vi "BNT_ULx-Content.vi"() -> (0 "CS++Classes & Messages":T1(array[cluster]))   [LabVIEW 2020]
doc: "Place actor and class constants that should be included included in the COMPACT application on the blockdiagramm."
uses:
  <vilib>/ActorFramework/Message/Message.lvclass
  BNT_ULx-MCSV/BNT_ULx-MCSV-I/BNT_ULx-MCSV-I/BNT_ULx-MCSV-I.lvclass
  C:/User/Brand/LVP/CSPP/CSPP-Template/Packages/CSPP_Core/Actors/CSPP_DeviceActor/CSPP_DeviceActor.lvclass
  CSPP_Core/Actors/CSPP_DeviceActor/CSPP_DeviceActor.lvclass
  C:/User/Brand/LVP/CSPP/CSPP-Template/Packages/CSPP_Core/Actors/CSPP_BaseActor/CSPP_BaseActor.lvclass
  CSPP_Core/Actors/CSPP_BaseActor/CSPP_BaseActor.lvclass
  BNT_ULx-MCSV/BNT_ULx-MCSV/BNT_ULx-MCSV.lvclass
  BNT_ULx-MCSV/BNT_ULx-MCSV-RTD/BNT_ULx-MCSV-RTD.lvclass
  BNT_ULx-MCSV/BNT_ULx-MCSV-TC/BNT_ULx-MCSV-TC.lvclass
  BNT_ULx-MCSV/BNT_ULx-MCSV-Ctr2Freq/BNT_ULx-MCSV-Ctr2Freq.lvclass
  BNT_ULx-MCSV/BNT_ULx-MCSV-DOPWM/BNT_ULx-MCSV-DOPWM.lvclass
  BNT_ULx-MCSV/BNT_ULx-MCSV-AIAvg/BNT_ULx-MCSV-AIAvg.lvclass
  C:/Program Files (x86)/National Instruments/LabVIEW 2020/vi.lib/ActorFramework/Actor/Actor.lvclass
  C:/User/Brand/LVP/CSPP/CSPP-Template/Packages/BNT_ULx/BNT_ULx-MCSV/BNT_ULx-MCSV/BNT_ULx-MCSV.lvclass
  C:/User/Brand/LVP/CSPP/CSPP-Template/Packages/BNT_ULx/BNT_ULx-MCSV/BNT_ULx-MCSV-RTD/BNT_ULx-MCSV-RTD.lvclass
  C:/User/Brand/LVP/CSPP/CSPP-Template/Packages/BNT_ULx/BNT_ULx-MCSV/BNT_ULx-MCSV-TC/BNT_ULx-MCSV-TC.lvclass
  C:/User/Brand/LVP/CSPP/CSPP-Template/Packages/BNT_ULx/BNT_ULx-MCSV/BNT_ULx-MCSV-Ctr2Freq/BNT_ULx-MCSV-Ctr2Freq.lvclass
  C:/User/Brand/LVP/CSPP/CSPP-Template/Packages/BNT_ULx/BNT_ULx-MCSV/BNT_ULx-MCSV-DOPWM/BNT_ULx-MCSV-DOPWM.lvclass
  C:/User/Brand/LVP/CSPP/CSPP-Template/Packages/BNT_ULx/BNT_ULx-MCSV/BNT_ULx-MCSV-AIAvg/BNT_ULx-MCSV-AIAvg.lvclass
  C:/User/Brand/LVP/CSPP/CSPP-Template/Packages/BNT_ULx/BNT_ULx-MCSV/BNT_ULx-MCSV-I/BNT_ULx-MCSV-I/BNT_ULx-MCSV-I.lvclass
panel:
  # "Place actor and class constants on the blockdiagramm."
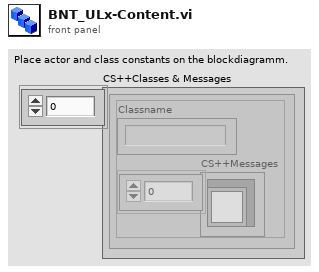
[diagram p1: front panel]
types:
  T1 = cluster{"Classname":string, "CS++Messages":refnum<class "Message.lvclass">[]}[]
  T2 = cluster{"class name":string, "CSPP_Messages":refnum<class "Message.lvclass">[]}
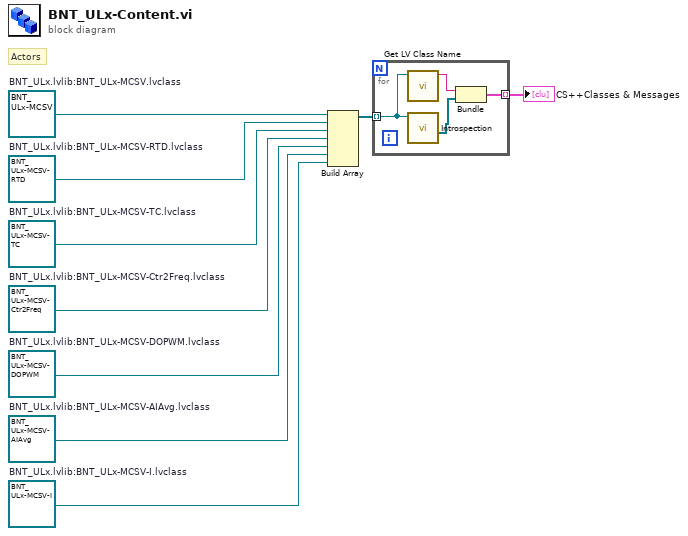
[diagram p0: block diagram]
diagram:
  w1 = refnum<class "BNT_ULx-MCSV-I.lvclass"> refnum  # BNT_ULx.lvlib:BNT_ULx-MCSV-I.lvclass
  w2 = refnum<class "BNT_ULx-MCSV-AIAvg.lvclass"> refnum  # BNT_ULx.lvlib:BNT_ULx-MCSV-AIAvg.lvclass
  w3 = refnum<class "BNT_ULx-MCSV-DOPWM.lvclass"> refnum  # BNT_ULx.lvlib:BNT_ULx-MCSV-DOPWM.lvclass
  w4 = refnum<class "BNT_ULx-MCSV-Ctr2Freq.lvclass"> refnum  # BNT_ULx.lvlib:BNT_ULx-MCSV-Ctr2Freq.lvclass
  w5 = refnum<class "BNT_ULx-MCSV-TC.lvclass"> refnum  # BNT_ULx.lvlib:BNT_ULx-MCSV-TC.lvclass
  w6 = refnum<class "BNT_ULx-MCSV-RTD.lvclass"> refnum  # BNT_ULx.lvlib:BNT_ULx-MCSV-RTD.lvclass
  w7 = refnum<class "BNT_ULx-MCSV.lvclass"> refnum  # BNT_ULx.lvlib:BNT_ULx-MCSV.lvclass
  # "Actors"
  n1 = Build Array(w7, w6, w5, w4, w3, w2, w1) -> (w9:refnum<class "BNT_ULx-MCSV.lvclass">[])
  n2 = for {
    tunnel: w9 -> [w13] mode=indexing
    tunnel: [w11] -> w8 mode=indexing
    n3 = call <vilib>:"Get LV Class Name.vi"("object"=w13) -> ("class name"=w12:string)  [unwired: 9 in, 1 out]
    n4 = call "Introspection.vi"("CSPP_BaseActor in"=w13) -> ("CSPP_Messages"=w10:refnum<class "Message.lvclass">[])  [unwired: 7 in, 3 out]
    n5 = Bundle("class name"=w12, "CSPP_Messages"=w10) -> (w11:T2)  [unwired: 1 in]
  }
  "CS++Classes & Messages" <- w8
